vi "Is leap year.vi"(8 "error in (no error)":errorcluster, 11 "Year":u32) -> (0 "error out":errorcluster, 2 "no. of days in year":u32, 3 "T = input is leap year":bool)   [LabVIEW 2021, in "Project Euler.lvlib"]
uses:
  Project Euler.lvlib
panel:
  # "Development\ncontrols/indicators useful for development and testing, but which are not outputs of the VI"
  # "Input\nInputs to the VI"
  # "Output\nOutputs of the VI"
  # "Description\n\nBlank VI with error handling case. \n\nSummarize the use of this VI in this space."
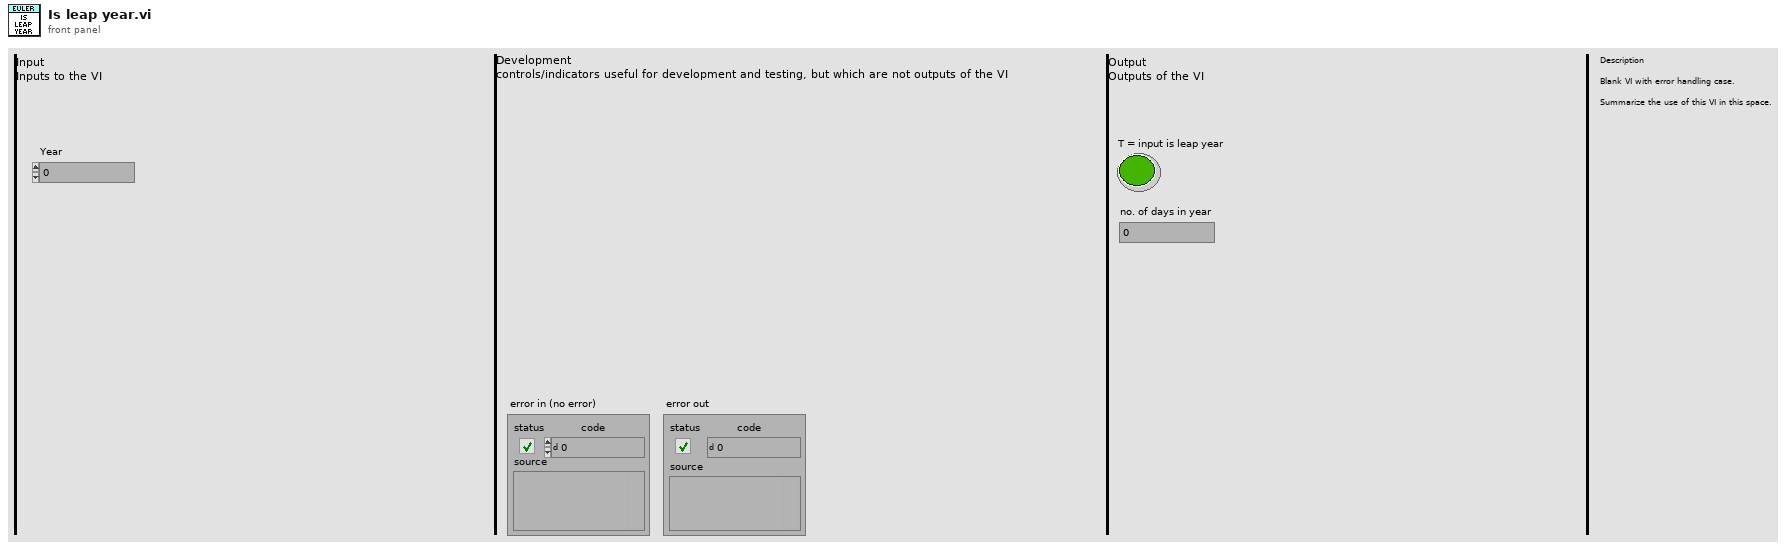
[diagram p1: front panel]
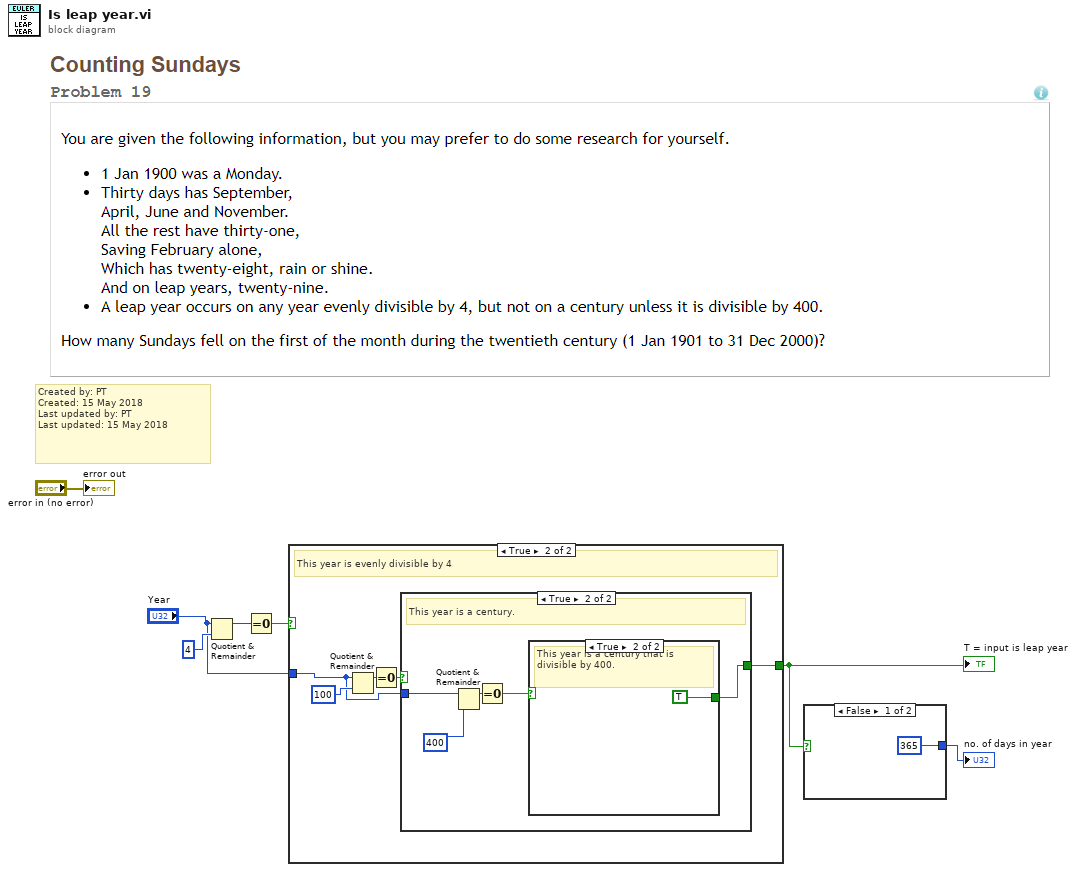
[diagram p0: block diagram]
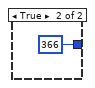
[diagram p2: hidden frame]
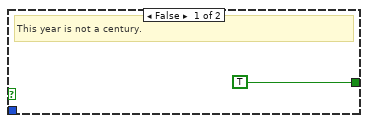
[diagram p4: hidden frame]
diagram:
  # "Created by: PT\nCreated: 15 May 2018\nLast updated by: PT\nLast updated: 15 May 2018"
  n1 = Quotient & Remainder(x="Year", y=u32 4) -> (x-y*floor(x/y)=w5:u32)  [unwired: 1 out]
  n2 = Equal To 0?(x=w5) -> (x = 0?=w4:bool)
  n3 = case shown="True" w4 {
    tunnel: "Year" -> [_ w8]
    tunnel: [_ w9] -> w2
    frame False {
      # "This year is not evenly divisible by 4."
    }
    frame True {
      # "This year is evenly divisible by 4"
      n4 = Quotient & Remainder(x=w8, y=u32 100) -> (x-y*floor(x/y)=w11:u32)  [unwired: 1 out]
      n5 = Equal To 0?(x=w11) -> (x = 0?=w10:bool)
      n6 = case shown="True" w10 {
        tunnel: [TRUE w14] -> w9
        tunnel: w8 -> [_ w16]
        frame False {
          # "This year is not a century."
        }
        frame True {
          # "This year is a century."
          n7 = Quotient & Remainder(x=w16, y=u32 400) -> (x-y*floor(x/y)=w18:u32)  [unwired: 1 out]
          n8 = Equal To 0?(x=w18) -> (x = 0?=w15:bool)
          n9 = case shown="True" w15 {
            tunnel: [_ TRUE] -> w14
            frame False {
              # "This year is a century that is NOT divisible by 400."
            }
            frame True {
              # "This year is a century that is divisible by 400."
            }
          }
        }
      }
    }
  }
  "T = input is leap year" <- w2
  n10 = case shown="False" w2 {
    tunnel: [u32 365 ("no. of days in year") u32 366 ("no. of days in year")] -> w1
    frame False {
    }
    frame True {
    }
  }
  "no. of days in year" <- w1
  "error out" <- "error in (no error)"
